vi "CommunicationTool-Ver1.vi"(0 "VISA资源名称":refnum<visa-resource-name>="COM29", 1 "SN":string, 2 "ModelNumber":string, 5 "通信协议名称":string, 7 "Slot":T1, 9 "DelayTime":u32=1000, 11 "error in":errorcluster, 12 "Debug":bool) -> (3 "字符串数值":bool, 4 "响应":string="ÿÿÿÿÿÿÿÿÿÿÿÿÿÿÿÿÿÿÿÿÿÿÿÿÿÿÿ", 6 "反馈结果":bool, 10 "CMD":string, 14 "data":string, 15 "error out":errorcluster)   [LabVIEW 2013]
doc: "本范例根据用户指示，对串口执行读写操作。范例运行时可按下“写入”或“读取”按钮，以及修改“读数”。\n\n设置的串口参数必须匹配连接仪器或设备的参数。本范例中，“读数”参数可指定串口读取的字节数。如端口字节超过指定的字节数，超出部分将不会被读取。如端口字节数少于指定的字节数，将返回超时错误。\n\n本范例可扩展流控制选项以包括XON和XOFF，从而允许用户选择控制字符。同时，用户可启用或禁用中止符。部分设备需要通过终止符确定命令字符串的结束位置。部分设备将发送终止符以说明待读取数据的末端。本范例演示了缓冲区中检测到终止符时，结束“读取”操作或添加终止符至“写入”数据末端的方法。"
uses:
  SystemCode/SysControl/Slot.ctl
  <vilib>/Utility/NIReport.llb/NI_report.lvclass
  SourceCode/PDINFO.ctl
  SourceCode/GlobalValue.vi
  <vilib>/Utility/error.llb/Error Cluster From Error Code.vi
  <vilib>/addons/_office/excel.llb/Excel Get Data ([str]).vi
  <vilib>/Utility/file.llb/Write To Spreadsheet File (string).vi
  <vilib>/Utility/file.llb/Read From Spreadsheet File (string).vi
  <vilib>/ErrorRing/Error Ring.xnode
  <vilib>/addons/_office/NI_ReportGenerationToolkit.lvlib
  <vilib>/Utility/NIReport.llb/Excel/NI_Excel.lvclass
panel:
  out "times":dbl
  out "反馈前段":string
  out "Time(ms)":u32
  out "SerNO":string
  out "硬件版本":string
  out "CCID":string="PASS"
  out "生产日期":string
  out "字符串":string
  out "x-y":u32
  out "读取缓冲区":string
  in  "命令列表":u16(ring)=17 items=["启动自动化测试", "退出自动化测试", "进入待机模式", "进入工作模式", "查询ACC IO状态", "GPS定位查询", "查询GPS定位时间", "GPS可见星数", "上网模块自检", "上网模块信号强度", "查询上网模块GPRS状态", "WIFI模块自检", "外部Flash测试", "查询电池电压", "查询电源电压", "CHARGE_CTL置低", "CHARGE_CTL置高", "查询CHARGE_WAKE状态", "3G_PWR_CTL输出低电平", "3G_PWR_CTL输出高电平", "3G_RST输出低电平", "3G_RST输出高电平", "查询ANT1_S状态", "查询ANT0_S状态", "GPS_PWREN输出低电平", "GPS_PWREN输出高电平", "CAN通信接收", "CAN通信发送", "重启", "U_CTL输出低电平", "U_CTL输出高电平", "OBD_CTL输出低电平", "OBD_CTL输出高电平", "OBD_STB输出低电平", "OBD_STB输出高电平", "3G_EN输出低电平", "3G_EN输出高电平", "写入主机条码", "读出主机条码", "写入生产日期", "读出生产日期", "读出CCID", "写入终端ID", "读出终端ID", "写入硬件版本", "读出硬件版本", "查看TBC文件", "进入休眠模式", "写入APN1", "写入APN2", "读出APN1", "读出APN2", "写入WIFI名称", "写入WIFI密码", "WIFI模块自检", "读出WIFI名称", "读出WIFI密码", "查询4G固件版本", "查询平台登录状态", "读OPEN软件版本", "写入车辆TUID", "读出车辆TUID", "查询MCU软件版本", "写入证书编号", "读出证书编号", "写入供应商代码", "读出供应商代码", "写入零部件号", "读出零部件号", "读出WIFI MAC地址", "OPEN模块自检", "切断备电供电", "恢复备电供电", "检测备电电压", "检测B+电源电压", "查询平台登录状态", "SRS碰撞检测", "读IMSI号", "读IMEI号"]
  out "Write":bool
  out "Read":bool
  out "ConfigPath":string="C:\\Users\\dell\\Desktop\\ExcelReport.vi"
  out "命令":string
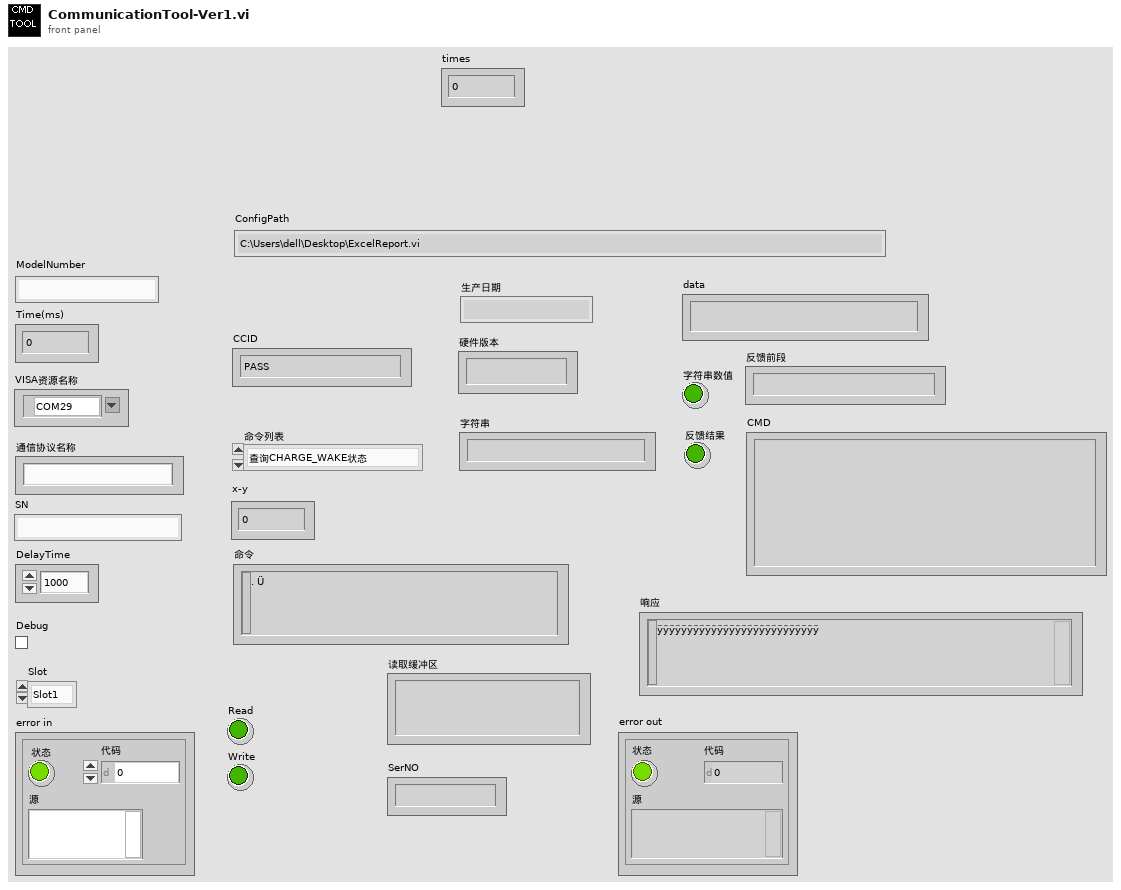
[diagram p1: front panel]
types:
  T1 = typedef "Slot.ctl" = enum16{"Slot1", "Slot2", "Slot3", "Slot4"}
  T2 = enum32{"invalid app kind", "Development System", "Run Time System", "Student Edition", "Embedded LabVIEW", "Evaluation", "Custom"}
  T3 = enum16{"maximized", "minimized", "normal", "no change"}
  T4 = enum16{"Standard Report", "HTML", "Word", "Excel"}
  T5 = typedef "PDINFO.ctl" = enum16{"Fw Ver", "HW Ver", "CCID", "WiFiName", "DevID", "SN", "TUID", "CertifID", "PdTime", "Provider", "WiFiPassword", "Imei", "AuthCode", "Reserved1", "Reserved2", "Reserved3"}
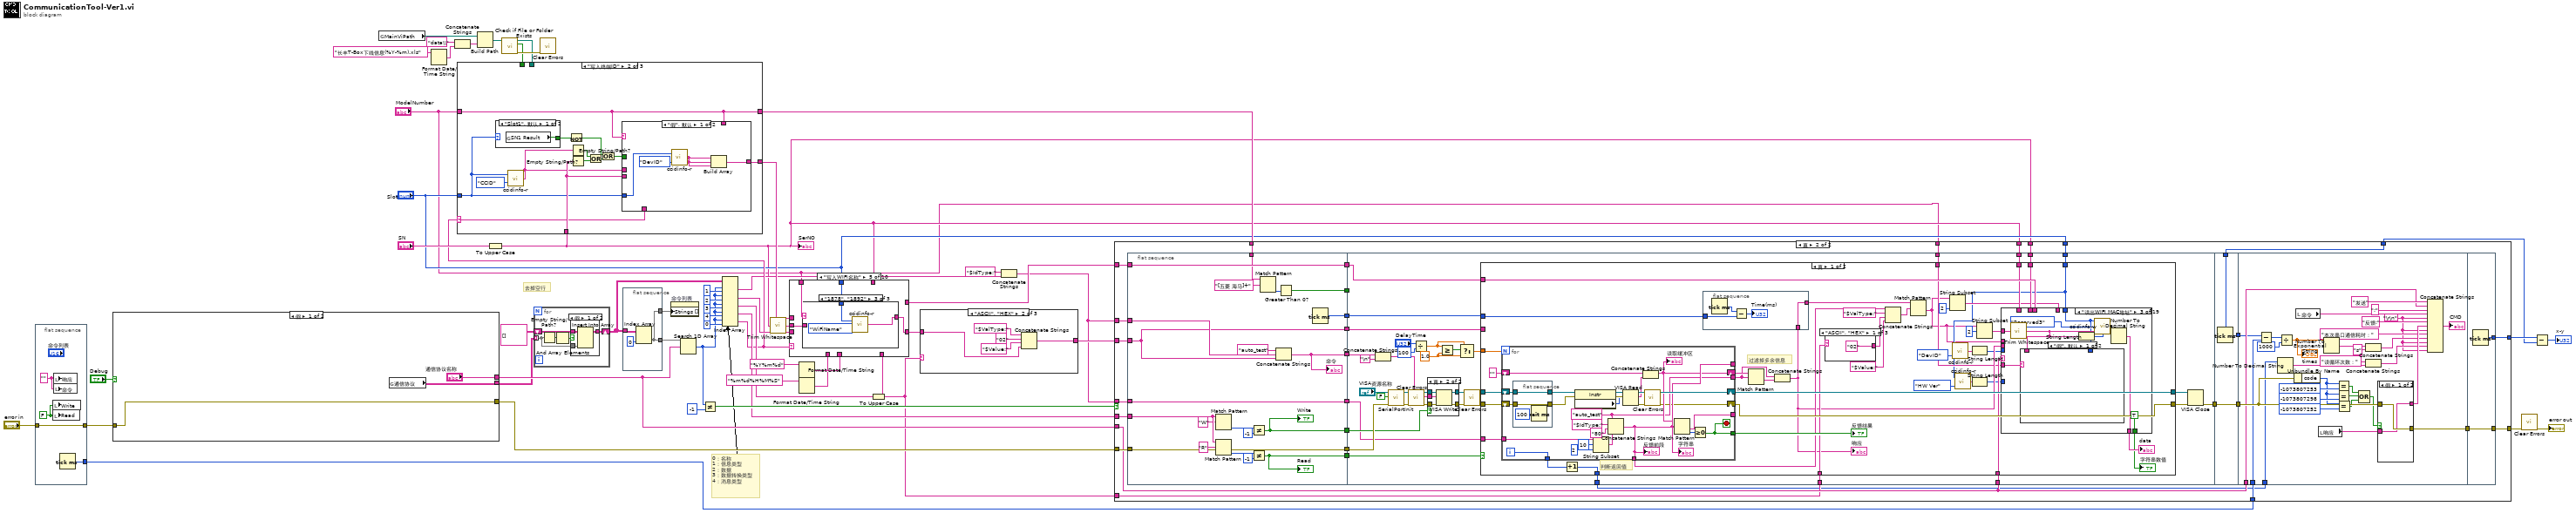
[diagram p0: block diagram]
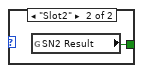
[diagram p3: hidden frame]
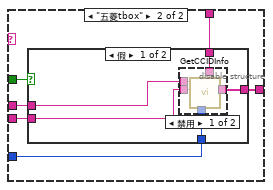
[diagram p4: hidden frame]
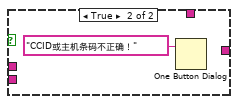
[diagram p6: hidden frame]
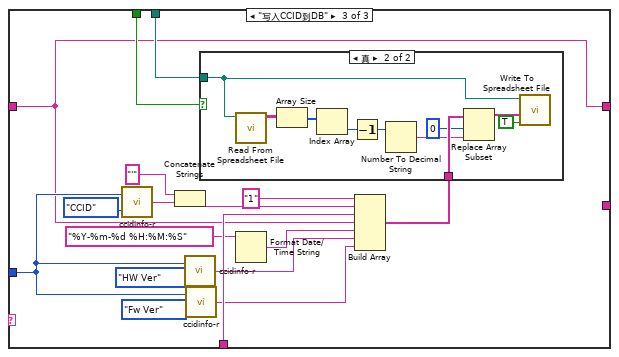
[diagram p7: hidden frame]
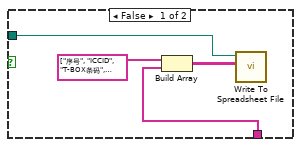
[diagram p8: hidden frame]
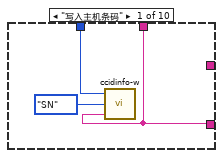
[diagram p9: hidden frame]
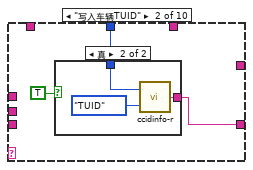
[diagram p10: hidden frame]
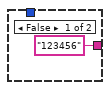
[diagram p11: hidden frame]
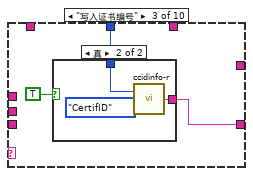
[diagram p12: hidden frame]
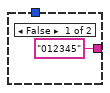
[diagram p13: hidden frame]
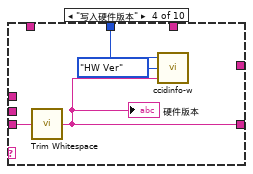
[diagram p14: hidden frame]
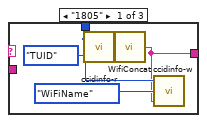
[diagram p15: hidden frame]
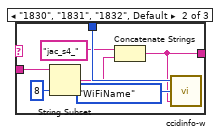
[diagram p16: hidden frame]
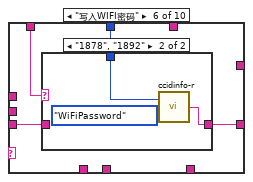
[diagram p17: hidden frame]
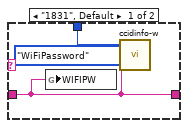
[diagram p18: hidden frame]
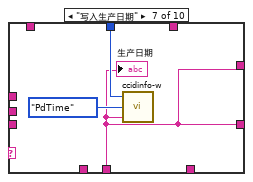
[diagram p19: hidden frame]
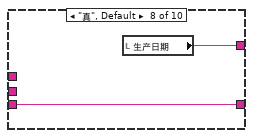
[diagram p20: hidden frame]
diagram:
  # "0：名称\n1：信息类型\n2：数据\n3：数据转换类型\n4：消息类型"
  # "去掉空行"
  n1 = flat-sequence {
    tunnel: "error in" -> [w57]
    tunnel: [w57] -> w53
    tunnel: [w56] -> w3
    frame #0 {
      w59 = FALSE ("Read")
      w58 = "" ("响应")
      n2 = local write "Write"(w59) -> ()
      n3 = local write "Read"(w59) -> ()
      n4 = local write "响应"(w58) -> ()
      n5 = local write "命令"(w58) -> ()
      n6 = Tick Count (ms)() -> (millisecond timer value=w56:u32)
    }
  }
  n7 = case shown="假" "Debug" {
    tunnel: [w61 w66] -> w51
    tunnel: w53 -> [w61 w65]
    tunnel: ["通信协议名称" w63] -> w44
    tunnel: [w60 w64] -> w19
    frame False {
      n8 = global read "GlobalValue.vi" "通信协议"() -> (w60:string[][])
    }
    frame True {
      n9 = property class="App"() -> ("App.Kind"=w75:T2)  [unwired: 2 in, 2 out]
      n10 = Equal?(x=T2."Run Time System" ("y"), y=w75) -> (x = y?=w77:bool)
      n11 = case shown="真" w77 {
        tunnel: [w111 w113] -> w76
        frame False {
          n12 = Current VI's Path() -> (path=w111:path)
        }
        frame True {
          n13 = Current VI's Path() -> (path=w112:path)
          n14 = Strip Path(path=w112) -> (stripped path=w113:path)  [unwired: 1 out]
        }
      }
      n15 = Strip Path(path=w76) -> (stripped path=w70:path)  [unwired: 1 out]
      n16 = Build Path(base path=w70, name or relative path="..\\config\\通信协议.xls" ("连接的字符串")) -> (appended path=w72:path)
      n17 = call <vilib>:"Check if File or Folder Exists.vi"("error in (no error)"=w65, "path"=w72) -> ("error out"=w67:errorcluster, "file or folder exists?"=w69:bool, "dup path"=w68:path)  [unwired: 7 out]
      n18 = Path To String(path=w72) -> (string=→"ConfigPath":string)
      n19 = case shown="假" w69 {
        tunnel: w68 -> [_ w88]
        tunnel: w67 -> [_ w87]
        tunnel: [w79 w86] -> w66
        tunnel: [_ w85] -> w64
        frame False {
          w80 = "通信协议.xls文件不存在!" ("消息")
          n20 = xnode "错误下拉列表"() -> ("错误输出"=w78:errorcluster)
          n21 = One Button Dialog(message=w80) -> ()  [unwired: 1 in, 1 out]
          n22 = Bundle By Name(cluster=w78, "source"=w80) -> (w79:errorcluster)
        }
        frame True {
          n23 = while {
            tunnel: w88 -> [w94]
            tunnel: [w93] -> w86
            tunnel: w87 -> [w92]
            shift-right: [w95] -> w85
            shift-left: _ -> [w90]
            stop <- TRUE stop-if-true
            n24 = First Call?() -> (First Call?: T/F=w89:bool)
            n25 = case shown="真" w89 {
              tunnel: [w97 w101] -> w95
              tunnel: w94 -> [_ w100]
              tunnel: [w96 w99] -> w93
              tunnel: w92 -> [w96 w98]
              tunnel: w90 -> [w97 _]
              frame False {
              }
              frame True {
                n26 = call <vilib>:"New Report.vi"("window state (normal)"=T3."no change", "report type"=T4."Excel", "template (empty)"=w100, "error in (no error)"=w98) -> ("report out"=w106:refnum<class "NI_report.lvclass">, "error out"=w107:errorcluster)  [unwired: 2 in, 8 out]
                n27 = call-poly <vilib>:"Excel Get Data.vi"("report in"=w106, "data type"=string[][] [], "error in (no error)"=w107) -> ("report out"=w103:refnum<class "NI_report.lvclass">, "data"=w108:string[][], "error out"=w102:errorcluster)  [unwired: 10 in]
                n28 = call-dynamic "Dispose Report.vi"("report in"=w103, "error in (no error)"=w102) -> ("error out"=w99:errorcluster)  [unwired: 3 in, 10 out]
                n29 = Delete From Array(array=w108, index (row)=0 ("索引 (行)")) -> (array with subset deleted=w101:string[][])  [unwired: 2 in, 1 out]
              }
            }
          }
        }
      }
      n30 = property on="命令列表" class="Ring (严格)"() -> ("RingText.Text"=w63:string)  [unwired: 2 in, 2 out]
    }
  }
  n31 = global read "GlobalValue.vi" "MainViPath"() -> (w25:path)
  n32 = Format Date/Time String(time format string (%c)="长丰T-Box下线信息(%Y-%m).xls" ("时间格式字符串(%c)")) -> (date/time string=w27:string)  [unwired: 2 in]
  n33 = Concatenate Strings("data\\" ("字符串"), w27) -> (w24:string)
  n34 = Build Path(base path=w25, name or relative path=w24) -> (appended path=w23:path)
  n35 = To Upper Case(1:"SN") -> (0:w9:string)
  "SerNO" <- w9
  n36 = call <vilib>:"Check if File or Folder Exists.vi"("path"=w23) -> ("error out"=w22:errorcluster, "file or folder exists?"=w20:bool, "dup path"=w21:path)  [unwired: 8 in]
  n37 = for {
    tunnel: w19 -> [w114] mode=indexing
    shift-right: [w117] -> w37
    shift-left: string[][] [] -> [w118]
    n38 = Empty String/Path?(string/path=w114) -> (empty?=w116:bool[])
    n39 = And Array Elements(Boolean array=w116) -> (logical AND=w115:bool)
    n40 = case shown="假" w115 {
      tunnel: w118 -> [w121 w122]
      tunnel: [w120 w122] -> w117
      tunnel: w114 -> [w119 _]
      frame False {
        n41 = Insert Into Array(array=w121, new element=w119) -> (w120:string[][])  [unwired: 2 in]
      }
      frame True {
      }
    }
  }
  n42 = call <vilib>:"Clear Errors.vi"("error in (no error)"=w22) -> ()  [unwired: 6 in, 1 out]
  n43 = flat-sequence {
    tunnel: [w123] -> w43
    tunnel: w37 -> [w124]
    tunnel: [w123] -> w16
    frame #0 {
      n44 = Index Array(array=w124, index (col)=0 ("禁用的索引 (列)")) -> (element=w123:string[])  [unwired: 1 in]
    }
  }
  n45 = property on="命令列表" class="Ring (严格)"("Strings []"=w16) -> ()  [unwired: 2 in, 2 out]
  n46 = Search 1D Array(1D array=w43, element=w44) -> (index of element=w15:i32)  [unwired: 1 in]
  n47 = Not Equal?(x=w15, y=-1) -> (x != y?=w46:bool)
  n48 = Index Array(array=w37, index (row) #1=w15, index (col) #1=1 ("索引 (列)"), index (row) #2=w15, index (col) #2=2 ("索引 (列)"), index (row) #3=w15, index (col) #3=3 ("索引 (列)"), index (row) #4=w15, index (col) #4=4 ("禁用的索引 (列)"), index (row) #5=w15, index (col) #5=0 ("禁用的索引 (列)")) -> (element #1=w12:string, element #2=w33:string, element #3=w39:string, element #4=w41:string, element #5=w14:string)
  n49 = case shown="\"写入终端ID\"" w14 {
    selector: w14 -> [_ w129 _]
    tunnel: [_ w139 _] -> w30
    tunnel: "ModelNumber" -> [w126 w128 w163]
    tunnel: w9 -> [_ w132 w178]
    tunnel: w21 -> [_ _ w174]
    tunnel: w20 -> [_ _ w173]
    tunnel: "Slot" -> [_ w127 w165]
    tunnel: [w126 w128 w163] -> w17
    frame "假", Default {
    }
    frame "写入终端ID" {
      n50 = case shown="\"Slot1\", 默认" w127 {
        tunnel: [w140 w141] -> w138
        frame "Slot1", Default {
          n51 = global read "GlobalValue.vi" "SN1 Result"() -> (w140:bool)
        }
        frame "Slot2" {
          n52 = global read "GlobalValue.vi" "SN2 Result"() -> (w141:bool)
        }
      }
      n53 = call "ccidinfo-r.vi"("Data Type"=PDINFO."CCID", "Slot"=w127) -> ("Data"=w130:string)
      n54 = Not(x=w138) -> (.not. x?=w135:bool)
      n55 = Empty String/Path?(string/path=w130) -> (empty?=w137:bool)
      n56 = Empty String/Path?(string/path=w132) -> (empty?=w136:bool)
      n57 = Or(x=w137, y=w136) -> (x .or. y?=w134:bool)
      n58 = Or(x=w135, y=w134) -> (x .or. y?=w133:bool)
      n59 = case shown="\"假\", 默认" w128 {
        tunnel: [w145 w151] -> w139
        tunnel: w133 -> [_ w150]
        tunnel: w128 -> [_ w149]
        tunnel: w132 -> [_ w148]
        tunnel: w127 -> [w143 w147]
        tunnel: w130 -> [_ w146]
        tunnel: w129 -> [_ _]
        frame "假", Default {
          n60 = call "ccidinfo-r.vi"("Data Type"=PDINFO."DevID", "Slot"=w143) -> ("Data"=w142:string)
          n61 = Build Array(w142, w142, w142) -> (w145:string[])
        }
        frame "五菱tbox" {
          n62 = case shown="假" w150 {
            tunnel: [w156 _] -> w151
            tunnel: w146 -> [w155 _]
            tunnel: w148 -> [w154 _]
            tunnel: w149 -> [w153 _]
            tunnel: w147 -> [w152 _]
            frame False {
              n63 = disable-structure shown="禁用" {
                disable-tunnel: [w161 _] -> w156
                disable-tunnel: w155 -> [w160 _]
                disable-tunnel: w154 -> [w159 _]
                disable-tunnel: w153 -> [w158 _]
                disable-tunnel: w152 -> [w157 _]
                frame Disabled {
                  n64 = call "GetCCIDInfo.vi"("table name"=w158, "Slot"=w157, "SerNO"=w159, "CCID"=w160) -> ("CCID信息"=w161:string[])  [unwired: 7 in]
                }
                frame Enabled {
                }
              }
            }
            frame True {
              n65 = One Button Dialog(message="CCID或主机条码不正确！" ("消息")) -> ()  [unwired: 1 in, 1 out]
            }
          }
        }
      }
    }
    frame "写入CCID到DB" {
      n66 = call "ccidinfo-r.vi"("Data Type"=PDINFO."CCID", "Slot"=w165) -> ("Data"=w169:string)
      n67 = Concatenate Strings("'", w169) -> (w171:string)
      n68 = call "ccidinfo-r.vi"("Data Type"=PDINFO."HW Ver", "Slot"=w165) -> ("Data"=w167:string)
      n69 = call "ccidinfo-r.vi"("Data Type"=PDINFO."Fw Ver", "Slot"=w165) -> ("Data"=w164:string)
      n70 = Format Date/Time String(time format string (%c)="%Y-%m-%d %H:%M:%S" ("时间格式字符串(%c)")) -> (date/time string=w176:string)  [unwired: 2 in]
      n71 = Build Array("1", w171, w178, w163, w176, w167, w164) -> (w175:string[])
      n72 = case shown="真" w173 {
        tunnel: w174 -> [w183 w184]
        tunnel: w175 -> [w182 w188]
        frame False {
          n73 = Build Array(string[] ["序号", "ICCID", "T-BOX条码", "设备型号", "生产日期", "硬件版本", "软件版本"], w182) -> (w181:string[][])
          n74 = call-poly <vilib>:"Write To Spreadsheet File.vi"("2D data"=w181, "file path (dialog if empty)"=w183) -> ()  [unwired: 6 in, 1 out]
        }
        frame True {
          n75 = call-poly <vilib>:"Read From Spreadsheet File.vi"("file path (dialog if empty)"=w184) -> ("all rows"=w193:string[][])  [unwired: 6 in, 4 out]
          n76 = Array Size(array=w193) -> (size(s)=w192:i32[])
          n77 = Index Array(array=w192) -> (element=w191:i32)  [unwired: 1 in]
          n78 = Decrement(x=w191) -> (x-1=w190:i32)
          n79 = Number To Decimal String(number=w190) -> (decimal integer string=w186:string)  [unwired: 1 in]
          n80 = Replace Array Subset(array=w188, new element=w186, index=0 ("索引")) -> (w185:string[])
          n81 = call-poly <vilib>:"Write To Spreadsheet File.vi"("append to file? (new file:F)"=TRUE, "1D data"=w185, "file path (dialog if empty)"=w184) -> ()  [unwired: 5 in, 1 out]
        }
      }
    }
  }
  n82 = call <vilib>:"Trim Whitespace.vi"("string"=w9) -> ("trimmed string"=w1:string)  [unwired: 1 in]
  n83 = Format Date/Time String(time format string (%c)="%Y%m%d" ("时间格式字符串(%c)")) -> (date/time string=w7:string)  [unwired: 2 in]
  n84 = Format Date/Time String(time format string (%c)="%m%d%H%M%S" ("时间格式字符串(%c)")) -> (date/time string=w5:string)  [unwired: 2 in]
  n85 = To Upper Case(1:w39) -> (0:w18:string)
  n86 = case shown="\"写入WIFI名称\"" w14 {
    tunnel: w33 -> [_ _ _ w212 _ w236 _ w248 w249 w252]
    tunnel: [w194 w199 w206 w211 w217 w235 w244 w248 w249 w252] -> w29
    tunnel: [_ _ _ _ _ _ w244 w247 _ _] -> w31
    tunnel: w9 -> [w194 _ _ _ _ _ _ _ _ _]
    tunnel: w1 -> [_ _ _ _ w215 _ _ _ _ _]
    tunnel: w30 -> [_ _ _ _ _ _ _ _ _ _]
    tunnel: "Slot" -> [w195 w198 w205 w214 w218 w237 w246 _ w251 w254]
    tunnel: w18 -> [_ _ _ _ _ _ _ _ _ _]
    tunnel: w7 -> [_ _ _ _ _ _ w244 _ _ _]
    tunnel: "ModelNumber" -> [_ _ _ _ w216 w234 _ _ _ _]
    tunnel: w5 -> [_ _ _ _ _ _ _ _ _ _]
    frame "写入主机条码" {
      n87 = call "ccidinfo-w.vi"("Data"=w194, "Data Type"=PDINFO."SN", "Slot"=w195) -> ()  [unwired: 1 in]
    }
    frame "写入车辆TUID" {
      n88 = case shown="真" TRUE {
        tunnel: ["123456" ("Data") w203] -> w199
        tunnel: w198 -> [_ w202]
        frame False {
        }
        frame True {
          n89 = call "ccidinfo-r.vi"("Data Type"=PDINFO."TUID", "Slot"=w202) -> ("Data"=w203:string)
        }
      }
    }
    frame "写入证书编号" {
      n90 = case shown="真" TRUE {
        tunnel: ["012345" ("Data") w210] -> w206
        tunnel: w205 -> [_ w209]
        frame False {
        }
        frame True {
          n91 = call "ccidinfo-r.vi"("Data Type"=PDINFO."CertifID", "Slot"=w209) -> ("Data"=w210:string)
        }
      }
    }
    frame "写入硬件版本" {
      n92 = call <vilib>:"Trim Whitespace.vi"("string"=w212) -> ("trimmed string"=w211:string)  [unwired: 1 in]
      "硬件版本" <- w211
      n93 = call "ccidinfo-w.vi"("Data"=w211, "Data Type"=PDINFO."HW Ver", "Slot"=w214) -> ()  [unwired: 1 in]
    }
    frame "写入WIFI名称" {
      n94 = case shown="\"1878\", \"1892\"" w216 {
        tunnel: w218 -> [w221 w229 w233]
        tunnel: [w219 w228 w231] -> w217
        tunnel: w215 -> [_ w226 _]
        frame "1805" {
          n95 = call "ccidinfo-r.vi"("Data Type"=PDINFO."TUID", "Slot"=w221) -> ("Data"=w220:string)
          n96 = call "WifiConcat.vi"("TUID"=w220) -> ("WIFIName"=w219:string)
          n97 = call "ccidinfo-w.vi"("Data"=w219, "Data Type"=PDINFO."WiFiName", "Slot"=w221) -> ()  [unwired: 1 in]
        }
        frame "1830", "1831", "1832", Default {
          n98 = String Subset(string=w226, length (rest)=8 ("长度（剩余）")) -> (substring=w224:string)  [unwired: 1 in]
          n99 = Concatenate Strings("jac_s4_" ("SerNO 2"), w224) -> (w228:string)
          n100 = call "ccidinfo-w.vi"("Data"=w228, "Data Type"=PDINFO."WiFiName", "Slot"=w229) -> ()  [unwired: 1 in]
        }
        frame "1878", "1892" {
          n101 = call "ccidinfo-r.vi"("Data Type"=PDINFO."WiFiName", "Slot"=w233) -> ("Data"=w231:string)
        }
      }
    }
    frame "写入WIFI密码" {
      n102 = case shown="\"1878\", \"1892\"" w234 {
        tunnel: w237 -> [w240 w242]
        tunnel: w236 -> [w238 _]
        tunnel: [w238 w241] -> w235
        frame "1831", Default {
          n103 = global write "GlobalValue.vi" "WIFIPW"(w238) -> ()
          n104 = call "ccidinfo-w.vi"("Data"=w238, "Data Type"=PDINFO."WiFiPassword", "Slot"=w240) -> ()  [unwired: 1 in]
        }
        frame "1878", "1892" {
          n105 = call "ccidinfo-r.vi"("Data Type"=PDINFO."WiFiPassword", "Slot"=w242) -> ("Data"=w241:string)
        }
      }
    }
    frame "写入生产日期" {
      n106 = call "ccidinfo-w.vi"("Data"=w244, "Data Type"=PDINFO."PdTime", "Slot"=w246) -> ()  [unwired: 1 in]
      "生产日期" <- w244
    }
    frame "真", Default {
      n107 = local read "生产日期"() -> (w247:string)
    }
    frame "写入供应商代码" {
      n108 = call "ccidinfo-w.vi"("Data"=w249, "Data Type"=PDINFO."Provider", "Slot"=w251) -> ()  [unwired: 1 in]
    }
    frame "写入零部件号" {
      n109 = call "ccidinfo-w.vi"("Data"=w252, "Data Type"=PDINFO."DevID", "Slot"=w254) -> ()  [unwired: 1 in]
    }
  }
  n110 = case shown="\"ASCII\", \"HEX\"" w18 {
    tunnel: [w255 w260 w265] -> w45
    tunnel: w29 -> [w256 w261 w266]
    frame "INT" {
      n111 = Concatenate Strings("$ValType:", "00", "$Value:", w256) -> (w255:string)
    }
    frame "ASCII", "HEX" {
      n112 = Concatenate Strings("$ValType:", "02", "$Value:", w261) -> (w260:string)
    }
    frame "STRING", Default {
      n113 = Concatenate Strings("$ValType:", "01", "$Value:", w266) -> (w265:string)
    }
  }
  n114 = Concatenate Strings("$IdType:", w12) -> (w11:string)
  n115 = case shown="真" w46 {
    tunnel: w44 -> [w274 w296]
    tunnel: w11 -> [_ w305]
    tunnel: w45 -> [_ w304]
    tunnel: w51 -> [_ w303]
    tunnel: [w270 w301] -> w55
    tunnel: w41 -> [_ w300]
    tunnel: w18 -> [_ w279]
    tunnel: [_ w292] -> w52
    tunnel: [_ w291] -> w36
    tunnel: w31 -> [_ w290]
    tunnel: w9 -> [_ w288]
    tunnel: w9 -> [_ w287]
    tunnel: "Slot" -> [_ w284]
    tunnel: w17 -> [_ w283]
    tunnel: w11 -> [_ w280]
    tunnel: "ModelNumber" -> [_ w278]
    tunnel: w3 -> [_ w276]
    frame False {
      (unwired) "FF" ("响应")
      n116 = Concatenate Strings(w274, "名称不存在" ("消息")) -> (w271:string)
      n117 = One Button Dialog(message=w271) -> ()  [unwired: 1 in, 1 out]
      n118 = Bundle By Name(cluster=errorcluster {"status"=TRUE, "code"=5000, "source"=""} ("error in 1 (no error)"), "source"=w271) -> (w270:errorcluster)
    }
    frame True {
      n119 = flat-sequence {
        tunnel: w305 -> [w315]
        tunnel: w304 -> [w313]
        tunnel: w303 -> [w326]
        tunnel: [w326] -> w302
        tunnel: w300 -> [w325]
        tunnel: [w318] -> w299
        tunnel: [w317] -> w298
        tunnel: [w316] -> w297
        tunnel: w290 -> [w314]
        tunnel: [w314] -> w289
        tunnel: [w313] -> w286
        tunnel: [w312] -> w285
        tunnel: w283 -> [w311]
        tunnel: [w308] -> w282
        tunnel: [w306] -> w281
        tunnel: w280 -> [w306]
        tunnel: w302 -> [w358]
        tunnel: w299 -> [w353]
        tunnel: w298 -> [w356]
        tunnel: [w357] -> w295
        tunnel: w297 -> [w336]
        tunnel: w296 -> [w344]
        tunnel: w289 -> [w343]
        tunnel: w288 -> [w342]
        tunnel: w287 -> [w341]
        tunnel: w286 -> [w340]
        tunnel: w285 -> [w339]
        tunnel: w284 -> [w338]
        tunnel: w282 -> [_]
        tunnel: w281 -> [w333]
        tunnel: w279 -> [w332]
        tunnel: w278 -> [w330]
        tunnel: [w329] -> w275
        tunnel: w295 -> [w644]
        tunnel: [w644] -> w294
        tunnel: [w643] -> w291
        tunnel: [w643] -> w277
        tunnel: w294 -> [w670]
        tunnel: w296 -> [w664]
        tunnel: [w671] -> w293
        tunnel: w277 -> [w658]
        tunnel: w276 -> [w657]
        tunnel: w275 -> [w650]
        tunnel: [w682] -> w301
        tunnel: w293 -> [w682]
        tunnel: [w681] -> w292
        frame #0 {
          n120 = Match Pattern(string=w325, regular expression="W" ("正则表达式")) -> (offset past match=w319:i32)  [unwired: 1 in, 3 out]
          n121 = Match Pattern(string=w325, regular expression="R" ("正则表达式")) -> (offset past match=w320:i32)  [unwired: 1 in, 3 out]
          n122 = Not Equal?(x=w319, y=-1) -> (x != y?=w318:bool)
          "Write" <- w318
          n123 = Not Equal?(x=w320, y=-1) -> (x != y?=w317:bool)
          "Read" <- w317
          n124 = Match Pattern(string=w311, regular expression="[五菱 海马]+" ("正则表达式")) -> (offset past match=w309:i32)  [unwired: 1 in, 3 out]
          n125 = Concatenate Strings("auto_test", w315, w313) -> (w316:string)
          "命令" <- w316
          n126 = Greater Than 0?(x=w309) -> (x > 0?=w308:bool)
          n127 = Tick Count (ms)() -> (millisecond timer value=w312:u32)
        }
        frame #1 {
          w350 = 1.0 ("y")
          n128 = Concatenate Strings(w336, "\n") -> (w334:string)
          n129 = call "SerialPortInit.vi"("错误输入"=w358, "海马"=FALSE, "COMIn"="VISA资源名称") -> ("错误输出"=w354:errorcluster, "COMOut"=w355:refnum<visa-resource-name>)  [unwired: 7 in]
          n130 = call <vilib>:"Clear Errors.vi"("error in (no error)"=w354) -> ("error out"=w328:errorcluster)  [unwired: 6 in]
          n131 = Divide(x="DelayTime", y=u32 100) -> (x/y=w349:dbl)
          n132 = case shown="真" w353 {
            tunnel: w355 -> [w362 w367]
            tunnel: [w362 w366] -> w352
            tunnel: [w361 w365] -> w351
            tunnel: w328 -> [w361 w364]
            tunnel: w334 -> [_ w363]
            frame False {
            }
            frame True {
              n133 = VISA Write(VISA resource name=w367, write buffer=w363, error in (no error)=w364) -> (VISA resource name out=w366:refnum<visa-resource-name>, error out=w365:errorcluster)  [unwired: 1 out]
            }
          }
          n134 = Greater Or Equal?(x=w349, y=w350) -> (x >= y?=w348:bool)
          n135 = Select(t=w349, s=w348, f=w350) -> (s? t:f=w345:dbl)
          n136 = call <vilib>:"Clear Errors.vi"("error in (no error)"=w351) -> ("error out"=w327:errorcluster)  [unwired: 6 in]
          n137 = case shown="真" w356 {
            tunnel: [w407 w642] -> w359
            tunnel: w352 -> [w406 w642]
            tunnel: [w408 w641] -> w360
            tunnel: w327 -> [w405 w641]
            tunnel: w345 -> [w403 _]
            tunnel: w344 -> [w402 _]
            tunnel: w343 -> [w399 _]
            tunnel: w342 -> [w398 _]
            tunnel: w341 -> [w397 _]
            tunnel: w340 -> [_ _]
            tunnel: w339 -> [w396 _]
            tunnel: w338 -> [w372 _]
            tunnel: w333 -> [w393 _]
            tunnel: w332 -> [w392 _]
            tunnel: w330 -> [w378 _]
            tunnel: [w376 _] -> w329
            frame True {
              # "过滤掉多余信息"
              # "判断返回值"
              n138 = for {
                N: w403 -> [_]
                shift-right: [w613] -> w408
                shift-left: w405 -> [w628]
                shift-right: [w616] -> w382
                shift-left: "" ("read buffer") -> [w632]
                shift-right: [w636] -> w407
                shift-left: w406 -> [w627]
                tunnel: [w626] -> w394
                tunnel: [w617] -> _
                tunnel: w393 -> [w624]
                tunnel: [w618] -> _
                tunnel: [w617] -> w391
                tunnel: [w615] -> w381
                tunnel: [w614] -> w377
                i -> [w614]
                stop <- w626 stop-if-true
                w615 = "auto_test"
                n139 = flat-sequence {
                  tunnel: w628 -> [w640]
                  tunnel: [w640] -> w629
                  tunnel: [w639] -> w630
                  tunnel: w627 -> [w639]
                  frame #0 {
                    n140 = Wait (ms)(milliseconds to wait=u32 100 ("等待时间（毫秒）")) -> ()  [unwired: 1 out]
                  }
                }
                n141 = property class="Instr"(reference=w630, error in=w629) -> (reference out=w635:refnum<visa-resource-name>, error out=w634:errorcluster, "Serial Settings:Number of Bytes at Serial Port"=w633:u32)
                n142 = String Subset(string=w624, offset (0)=10 ("偏移量(0)"), length (rest)=2 ("长度（剩余）")) -> (substring=w625:string)
                n143 = Concatenate Strings(w615, "$IdType:", "80" ("字符串"), w625) -> (w617:string)
                "字符串" <- w617
                "反馈前段" <- w617
                n144 = VISA Read(VISA resource name=w635, byte count=w633, error in (no error)=w634) -> (VISA resource name out=w636:refnum<visa-resource-name>, read buffer=w631:string, error out=w637:errorcluster)  [unwired: 1 out]
                n145 = Concatenate Strings(w632, w631) -> (w616:string)
                "读取缓冲区" <- w616
                n146 = call <vilib>:"Clear Errors.vi"("error in (no error)"=w637) -> ("error out"=w613:errorcluster)  [unwired: 6 in]
                n147 = Match Pattern(string=w616, regular expression=w617) -> (after substring=w618:string, offset past match=w619:i32)  [unwired: 1 in, 2 out]
                n148 = Greater Or Equal To 0?(x=w619) -> (x >= 0?=w626:bool)
              }
              "反馈结果" <- w394
              n149 = Increment(x=w377) -> (x+1=w376:i32)
              n150 = flat-sequence {
                tunnel: w396 -> [w610]
                tunnel: w379 -> [w609]
                tunnel: [w609] -> w395
                frame #0 {
                  n151 = Tick Count (ms)() -> (millisecond timer value=w611:u32)
                  n152 = Subtract(x=w611, y=w610) -> (x-y=→"Time(ms)":u32)
                }
              }
              n153 = Match Pattern(string=w382, regular expression=w381) -> (after substring=w380:string)  [unwired: 1 in, 3 out]
              n154 = Concatenate Strings(w381, w380) -> (w379:string)
              "响应" <- w379
              n155 = case shown="\"ASCII\", \"HEX\"" w392 {
                tunnel: ["02" "01" "00"] -> w389
                frame "ASCII", "HEX" {
                }
                frame "STRING", Default {
                }
                frame "INT" {
                }
              }
              n156 = Concatenate Strings(w391, "$ValType:", w389, "$Value:") -> (w387:string)
              n157 = Match Pattern(string=w395, regular expression=w387) -> (after substring=w368:string)  [unwired: 1 in, 3 out]
              n158 = String Subset(string=w368, length (rest)=2) -> (substring=w385:string)  [unwired: 1 in]
              n159 = call "ccidinfo-r.vi"("Data Type"=PDINFO."DevID", "Slot"=w372) -> ("Data"=w374:string)
              n160 = call "ccidinfo-r.vi"("Data Type"=PDINFO."HW Ver", "Slot"=w372) -> ("Data"=w370:string)
              n161 = String Length(string=w374) -> (length=w373:i32)
              n162 = String Length(string=w370) -> (length=w369:i32)
              n163 = String Subset(string=w368, offset (0)=2) -> (substring=w383:string)  [unwired: 1 in]
              n164 = case shown="\"读出WIFI MAC地址\"" w402 {
                tunnel: [w413 w417 w425 w443 w453 w463 w473 w486 w502 w510 w520 w535 w546 w557 w566 w571 w585 w595 w607] -> w401
                tunnel: [FALSE FALSE TRUE FALSE FALSE FALSE FALSE FALSE FALSE FALSE FALSE FALSE FALSE FALSE FALSE FALSE FALSE TRUE TRUE] -> w400
                tunnel: w385 -> [w414 _ _ _ _ _ _ _ _ _ _ w529 _ _ _ _ _ _ _]
                tunnel: w399 -> [_ _ _ _ _ _ _ _ _ _ _ _ _ _ _ _ _ _ _]
                tunnel: w398 -> [_ _ _ _ _ _ _ _ _ _ _ _ _ _ _ _ _ _ _]
                tunnel: w397 -> [_ _ _ _ _ _ _ _ _ _ _ _ _ _ _ _ _ _ _]
                tunnel: w372 -> [_ _ w421 w441 w451 w461 w471 w484 w499 w506 w519 w534 w545 w556 w564 w573 w582 _ _]
                tunnel: w379 -> [_ _ _ _ _ _ _ _ _ _ _ _ _ _ _ _ _ _ _]
                tunnel: w383 -> [_ w418 w424 w442 w452 w462 w472 w485 w497 w509 w516 w531 _ _ w565 w572 w584 w597 w608]
                tunnel: w378 -> [_ _ w420 _ _ _ _ w479 _ _ _ _ _ _ _ _ w577 w594 _]
                tunnel: w373 -> [_ _ _ _ _ _ _ w478 _ _ _ _ _ _ _ _ _ _ _]
                tunnel: w369 -> [_ _ _ _ _ _ _ _ _ _ _ _ _ _ _ _ w576 _ _]
                tunnel: w368 -> [_ _ _ _ _ _ _ _ _ _ _ _ w540 w551 _ _ _ _ _]
                frame "真", Default {
                  n165 = Empty String/Path?(string/path=w414) -> (empty?=w415:bool)
                  n166 = Select(t="", s=w415, f=w414) -> (s? t:f=w413:string)
                }
                frame "E-call状态返回", "查询4G固件版本", "读OPEN软件版本" {
                  n167 = call <vilib>:"Trim Whitespace.vi"("string"=w418) -> ("trimmed string"=w417:string)  [unwired: 1 in]
                }
                frame "读出WIFI MAC地址" {
                  n168 = call <vilib>:"Trim Whitespace.vi"("string"=w424) -> ("trimmed string"=w422:string)  [unwired: 1 in]
                  n169 = case shown="\"假\", 默认" w420 {
                    tunnel: w422 -> [_ w437]
                    tunnel: w421 -> [_ w430]
                    frame "假", Default {
                    }
                    frame "1878", "1892" {
                      n170 = call "StrChange.vi"("StrIn"=w437) -> ("StrOut"=w433:string)  [unwired: 9 in, 1 out]
                      n171 = call "StrToPW.vi"("StrIn"=w433) -> ("StrOut"=w431:string)  [unwired: 9 in, 1 out]
                      n172 = Concatenate Strings("Hotspot" ("字符串"), w433) -> (w435:string)
                      n173 = Concatenate Strings("jmsg" ("字符串"), w431) -> (w428:string)
                      n174 = call "ccidinfo-w.vi"("Data"=w435, "Data Type"=PDINFO."WiFiName", "Slot"=w430) -> ()  [unwired: 1 in]
                      n175 = call "ccidinfo-w.vi"("Data"=w428, "Data Type"=PDINFO."WiFiPassword", "Slot"=w430) -> ()  [unwired: 1 in]
                    }
                  }
                  n176 = String Length(string=w422) -> (length=w426:i32)
                  n177 = call "ccidinfo-w.vi"("Data"=w422, "Data Type"=PDINFO."Reserved3", "Slot"=w421) -> ()  [unwired: 1 in]
                  n178 = Number To Decimal String(number=w426) -> (decimal integer string=w425:string)  [unwired: 1 in]
                }
                frame "读出主机条码" {
                  n179 = call <vilib>:"Trim Whitespace.vi"("string"=w442) -> ("trimmed string"=w438:string)  [unwired: 1 in]
                  n180 = call "ccidinfo-r.vi"("Data Type"=PDINFO."SN", "Slot"=w441) -> ("Data"=w439:string)
                  n181 = Equal?(x=w438, y=w439) -> (x = y?=w446:bool)
                  n182 = Select(t="PASS" ("string"), s=w446, f="FAIL") -> (s? t:f=w443:string)
                }
                frame "读出车辆TUID" {
                  n183 = call <vilib>:"Trim Whitespace.vi"("string"=w452) -> ("trimmed string"=w448:string)  [unwired: 1 in]
                  n184 = call "ccidinfo-r.vi"("Data Type"=PDINFO."TUID", "Slot"=w451) -> ("Data"=w449:string)
                  n185 = Equal?(x=w448, y=w449) -> (x = y?=w456:bool)
                  n186 = Select(t="PASS" ("string"), s=w456, f="FAIL") -> (s? t:f=w453:string)
                }
                frame "读出证书编号" {
                  n187 = call <vilib>:"Trim Whitespace.vi"("string"=w462) -> ("trimmed string"=w458:string)  [unwired: 1 in]
                  n188 = call "ccidinfo-r.vi"("Data Type"=PDINFO."CertifID", "Slot"=w461) -> ("Data"=w459:string)
                  n189 = Equal?(x=w458, y=w459) -> (x = y?=w466:bool)
                  n190 = Select(t="PASS" ("string"), s=w466, f="FAIL") -> (s? t:f=w463:string)
                }
                frame "读出供应商代码" {
                  n191 = call <vilib>:"Trim Whitespace.vi"("string"=w472) -> ("trimmed string"=w468:string)  [unwired: 1 in]
                  n192 = call "ccidinfo-r.vi"("Data Type"=PDINFO."Provider", "Slot"=w471) -> ("Data"=w469:string)
                  n193 = Equal?(x=w468, y=w469) -> (x = y?=w476:bool)
                  n194 = Select(t="PASS" ("string"), s=w476, f="FAIL") -> (s? t:f=w473:string)
                }
                frame "读出零部件号" {
                  n195 = call <vilib>:"Trim Whitespace.vi"("string"=w485) -> ("trimmed string"=w481:string)  [unwired: 1 in]
                  n196 = case shown="\"1805\"" w479 {
                    tunnel: w481 -> [w491 w494]
                    tunnel: [w491 w493] -> w480
                    tunnel: w478 -> [_ w492]
                    frame "1805" {
                    }
                    frame "1830", "1831", "1832", Default {
                      n197 = String Subset(string=w494, length (rest)=w492) -> (substring=w493:string)  [unwired: 1 in]
                    }
                  }
                  n198 = call "ccidinfo-r.vi"("Data Type"=PDINFO."DevID", "Slot"=w484) -> ("Data"=w482:string)
                  n199 = Equal?(x=w480, y=w482) -> (x = y?=w489:bool)
                  n200 = Select(t="PASS" ("string"), s=w489, f="FAIL") -> (s? t:f=w486:string)
                }
                frame "读出WIFI名称" {
                  n201 = call <vilib>:"Trim Whitespace.vi"("string"=w497) -> ("trimmed string"=w495:string)  [unwired: 1 in]
                  n202 = call "ccidinfo-r.vi"("Data Type"=PDINFO."WiFiName", "Slot"=w499) -> ("Data"=w498:string)
                  n203 = Equal?(x=w495, y=w498) -> (x = y?=w501:bool)
                  n204 = Select(t="PASS" ("string"), s=w501, f="FAIL") -> (s? t:f=w502:string)
                }
                frame "读出WIFI密码" {
                  w505 = PDINFO."WiFiPassword" ("Data Type")
                  n205 = call <vilib>:"Trim Whitespace.vi"("string"=w509) -> ("trimmed string"=w508:string)  [unwired: 1 in]
                  n206 = call "ccidinfo-r.vi"("Data Type"=w505, "Slot"=w506) -> ("Data"=w507:string)
                  n207 = call "ccidinfo-w.vi"("Data"=w508, "Data Type"=w505, "Slot"=w506) -> ()  [unwired: 1 in]
                  n208 = Equal?(x=w508, y=w507) -> (x = y?=w513:bool)
                  n209 = Select(t="PASS" ("string"), s=w513, f="FAIL") -> (s? t:f=w510:string)
                }
                frame "读出CCID" {
                  n210 = call <vilib>:"Trim Whitespace.vi"("string"=w516) -> ("trimmed string"=w515:string)  [unwired: 1 in]
                  n211 = String Length(string=w515) -> (length=w523:i32)
                  n212 = Equal?(x=w523, y=20) -> (x = y?=w521:bool)
                  n213 = To Upper Case(1:w515) -> (0:w517:string)
                  "CCID" <- w517
                  n214 = Select(t="PASS" ("string"), s=w521, f="FAIL") -> (s? t:f=w520:string)
                  n215 = call "ccidinfo-w.vi"("Data"=w517, "Data Type"=PDINFO."CCID", "Slot"=w519) -> ()  [unwired: 1 in]
                }
                frame "读取IMSI号" {
                  n216 = call <vilib>:"Trim Whitespace.vi"("string"=w531) -> ("trimmed string"=w530:string)  [unwired: 1 in]
                  n217 = Equal?(x=w529, y="01") -> (x = y?=w527:bool)
                  n218 = To Upper Case(1:w530) -> (0:w532:string)
                  n219 = Select(t="PASS" ("string"), s=w527, f="FAIL") -> (s? t:f=w535:string)
                  n220 = call "ccidinfo-w.vi"("Data"=w532, "Data Type"=PDINFO."Imei", "Slot"=w534) -> ()  [unwired: 1 in]
                }
                frame "读IMSI号" {
                  n221 = call <vilib>:"Trim Whitespace.vi"("string"=w540) -> ("trimmed string"=w539:string)  [unwired: 1 in]
                  n222 = String Length(string=w539) -> (length=w542:i32)
                  n223 = Equal?(x=w542, y=15) -> (x = y?=w543:bool)
                  n224 = Select(t="PASS" ("string"), s=w543, f="FAIL") -> (s? t:f=w546:string)
                  n225 = call "ccidinfo-w.vi"("Data"=w539, "Data Type"=PDINFO."AuthCode", "Slot"=w545) -> ()  [unwired: 1 in]
                }
                frame "读IMEI号" {
                  n226 = call <vilib>:"Trim Whitespace.vi"("string"=w551) -> ("trimmed string"=w550:string)  [unwired: 1 in]
                  n227 = String Length(string=w550) -> (length=w553:i32)
                  n228 = Equal?(x=w553, y=15) -> (x = y?=w554:bool)
                  n229 = Select(t="PASS" ("string"), s=w554, f="FAIL") -> (s? t:f=w557:string)
                  n230 = call "ccidinfo-w.vi"("Data"=w550, "Data Type"=PDINFO."Imei", "Slot"=w556) -> ()  [unwired: 1 in]
                }
                frame "读出生产日期" {
                  n231 = call <vilib>:"Trim Whitespace.vi"("string"=w565) -> ("trimmed string"=w561:string)  [unwired: 1 in]
                  n232 = call "ccidinfo-r.vi"("Data Type"=PDINFO."PdTime", "Slot"=w564) -> ("Data"=w562:string)
                  n233 = Equal?(x=w561, y=w562) -> (x = y?=w569:bool)
                  n234 = Select(t="PASS" ("string"), s=w569, f="FAIL") -> (s? t:f=w566:string)
                }
                frame "查询MCU软件版本" {
                  n235 = call <vilib>:"Trim Whitespace.vi"("string"=w572) -> ("trimmed string"=w571:string)  [unwired: 1 in]
                  n236 = call "ccidinfo-w.vi"("Data"=w571, "Data Type"=PDINFO."Fw Ver", "Slot"=w573) -> ()  [unwired: 1 in]
                }
                frame "读出硬件版本" {
                  n237 = call <vilib>:"Trim Whitespace.vi"("string"=w584) -> ("trimmed string"=w580:string)  [unwired: 1 in]
                  n238 = case shown="\"1830\", \"1831\", \"1832\", 默认" w577 {
                    tunnel: w580 -> [w590 w593]
                    tunnel: [w590 w592] -> w578
                    tunnel: w576 -> [_ w591]
                    frame "1805" {
                    }
                    frame "1830", "1831", "1832", Default {
                      n239 = String Subset(string=w593, length (rest)=w591) -> (substring=w592:string)  [unwired: 1 in]
                    }
                  }
                  n240 = call "ccidinfo-r.vi"("Data Type"=PDINFO."HW Ver", "Slot"=w582) -> ("Data"=w581:string)
                  n241 = call <vilib>:"Trim Whitespace.vi"("string"=w581) -> ("trimmed string"=w579:string)  [unwired: 1 in]
                  n242 = Equal?(x=w578, y=w579) -> (x = y?=w588:bool)
                  n243 = Select(t="PASS" ("string"), s=w588, f="FAIL") -> (s? t:f=w585:string)
                }
                frame "检测B+电源电压", "检测备电电压" {
                  n244 = case shown="\"1805\"" w594 {
                    tunnel: w597 -> [w604 w605]
                    tunnel: [w599 w605] -> w595
                    frame "1805" {
                      n245 = call <vilib>:"Trim Whitespace.vi"("string"=w604) -> ("trimmed string"=w603:string)  [unwired: 1 in]
                      n246 = String To Byte Array(string=w603) -> (unsigned byte array=w602:u8[])
                      n247 = Index Array(array=w602) -> (element=w600:u8)  [unwired: 1 in]
                      n248 = Divide(x=w600, y=10) -> (x/y=w598:dbl)
                      n249 = Number To Fractional String(number=w598) -> (F-format string=w599:string)  [unwired: 3 in]
                    }
                    frame "1830", "1831", "1832", Default {
                    }
                  }
                }
                frame "上网模块信号强度" {
                  n250 = call <vilib>:"Trim Whitespace.vi"("string"=w608) -> ("trimmed string"=w607:string)  [unwired: 1 in]
                }
              }
              "data" <- w401
              "字符串数值" <- w400
            }
            frame False {
            }
          }
          n251 = VISA Close(VISA resource name=w359, error in (no error)=w360) -> (error out=w357:errorcluster)
        }
        frame #2 {
          n252 = Tick Count (ms)() -> (millisecond timer value=w643:u32)
        }
        frame #3 {
          w645 = "\r\n"
          n253 = Subtract(x=w658, y=w657) -> (x-y=w656:u32)
          n254 = Number To Decimal String(number=w650) -> (decimal integer string=w647:string)  [unwired: 1 in]
          n255 = Divide(x=w656, y=1000) -> (x/y=w654:dbl)
          "times" <- w654
          n256 = Unbundle By Name(w670) -> ("code"=w667:i32)
          n257 = local read "命令"() -> (w659:string)
          n258 = local read "响应"() -> (w665:string)
          n259 = Number To Exponential String(number=w654) -> (E-format string=w652:string)  [unwired: 3 in]
          n260 = Equal?(x=w667, y=-1073807253) -> (x = y?=w663:bool)
          n261 = Equal?(x=w667, y=-1073807298) -> (x = y?=w662:bool)
          n262 = Equal?(x=w667, y=-1073807252) -> (x = y?=w661:bool)
          n263 = Compound Arithmetic op=OR(w663, w662, w661) -> (w660:bool)
          n264 = Concatenate Strings(w652, "s") -> (w651:string)
          n265 = Concatenate Strings("读循环次数：" ("字符串"), w647) -> (w646:string)
          n266 = case shown="假" w660 {
            tunnel: [w678 errorcluster {"status"=FALSE, "code"=0, "source"=""} ("t")] -> w671
            tunnel: w670 -> [w678 _]
            tunnel: w665 -> [w677 _]
            tunnel: [w677 ""] -> w669
            frame False {
            }
            frame True {
            }
          }
          n267 = Concatenate Strings("发送" ("字符串"), w664, ":" ("字符串"), w659, w645, "反馈:" ("字符串"), w669, w645, "本次串口通信耗时：", w651, w645, w646, w645) -> (→"CMD":string)
        }
        frame #4 {
          n268 = Tick Count (ms)() -> (millisecond timer value=w681:u32)
        }
      }
    }
  }
  n269 = call <vilib>:"Clear Errors.vi"("error in (no error)"=w55) -> ("error out"=→"error out":errorcluster)  [unwired: 6 in]
  n270 = Subtract(x=w52, y=w36) -> (x-y=→"x-y":u32)
